vi "Filter Only Eulogy.vi"(8 "Error In":errorcluster, 11 "VI Bookmarks":T1[](array[typedef])) -> (0 "Error Out":errorcluster, 3 "Eulogy Bookmarks":T1[](array[typedef]))   [LabVIEW 2017, in "Bookmark Manager.lvlib"]
doc: "Filters out all bookmarks that are NOT graves"
uses:
  Bookmark Manager.lvlib
  Controls/VI Bookmark.ctl
  Controls/VI Information.ctl
  Controls/Application Information.ctl
  Toolkit VIs/Public/Typedefs/Bookmarks.ctl
  Toolkit VIs/Toolkit VIs.lvlib
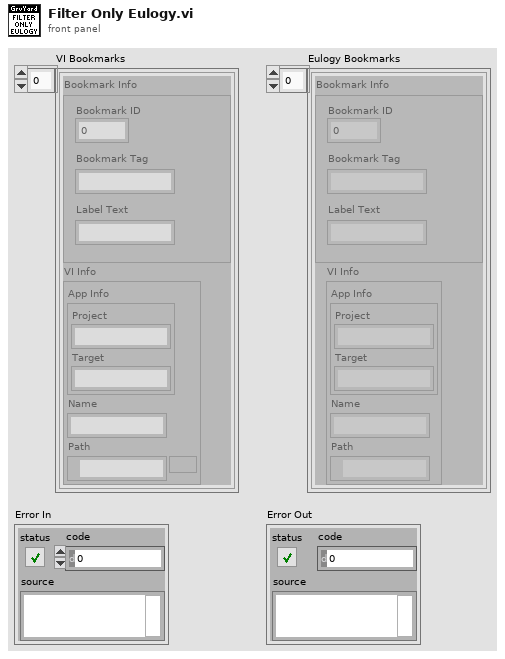
[diagram p1: front panel]
types:
  T1 = typedef "Bookmark Manager.lvlib/VI Bookmark.ctl" = cluster{"Bookmark Info":cluster{"Bookmark ID":u32, "Bookmark Tag":string, "Label Text":string}, "VI Info":T2}
  T2 = typedef "Bookmark Manager.lvlib/VI Information.ctl" = cluster{"App Info":T3, "Name":string, "Path":path}
  T3 = typedef "Bookmark Manager.lvlib/Application Information.ctl" = cluster{"Project":string, "Target":string}
  T4 = typedef "Toolkit VIs.lvlib/Bookmarks.ctl" = enum16{"RIP", "Zombie"}
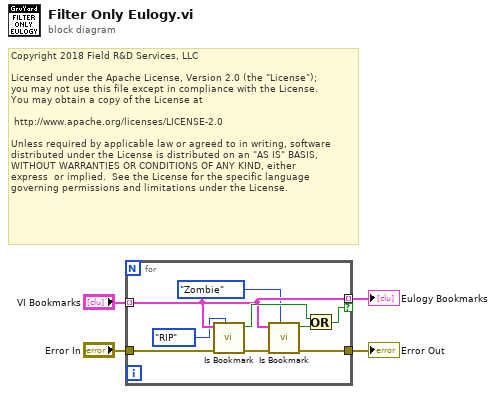
[diagram p0: block diagram]
diagram:
  # "Copyright 2018 Field R&D Services, LLC\n\nLicensed under the Apache License, Version 2.0 (the \"License\");\nyou may not use this file except in compliance with the License.\nYou may obtain a copy of the License at\n\n\thttp://www.apache.org/licenses/LICENSE-2.0\n\nUnless required by applicable law or agreed to in writing, software\ndistributed under the License is distributed on an \"AS IS\" BASIS,\nWITHOUT WARRANTIES OR CONDITIONS OF ANY KIND, either \nexpress  or implied.  See the License for the specific language \ngoverning permissions and limitations under the License."
  n1 = for {
    tunnel: "VI Bookmarks" -> [w10] mode=indexing
    tunnel: [w10] -> w1 mode=indexing if=w13
    tunnel: "Error In" -> [w9]
    tunnel: [w7] -> w3
    n2 = call "Is Bookmark.vi"("Bookmark"=Bookmarks."RIP", "Error In"=w9, "VI Bookmark"=w10) -> ("Error Out"=w8:errorcluster, "Is Bookmark"=w11:bool)  [unwired: 7 in]
    n3 = call "Is Bookmark.vi"("Bookmark"=Bookmarks."Zombie", "Error In"=w8, "VI Bookmark"=w10) -> ("Error Out"=w7:errorcluster, "Is Bookmark"=w12:bool)  [unwired: 7 in]
    n4 = Or(x=w11, y=w12) -> (x .or. y?=w13:bool)
  }
  "Error Out" <- w3
  "Eulogy Bookmarks" <- w1
